vi "Destroy User Events.vi"(11 "EDS Viewer in":refnum<class "EDS Viewer.lvclass">) -> (3 "EDS Viewer out":refnum<class "EDS Viewer.lvclass">)   [LabVIEW 2024, in "EDS Viewer.lvlib" / "EDS Viewer.lvclass"]
uses:
  EDS Viewer.lvclass
  EDS Viewer.lvclass/EDS Viewer.ctl
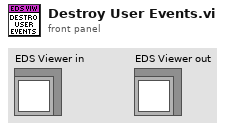
[diagram p1: front panel]
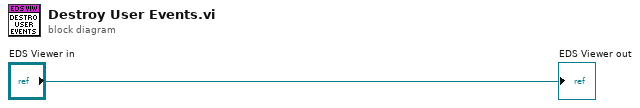
[diagram p0: block diagram]
diagram:
  "EDS Viewer out" <- "EDS Viewer in"
